vi "一体站流程自动启动.vi"(11 "参数":T1) -> ()   [LabVIEW 2016, in "PLC.lvlib"]
uses:
  PLC.lvlib
  <vilib>/ptbypt/NI_PtbyPt.lvlib
panel:
  out "s? t:f":enum16{"初始化", "采配水启动", "仪器操作", "反冲洗", "结束"}(ring)
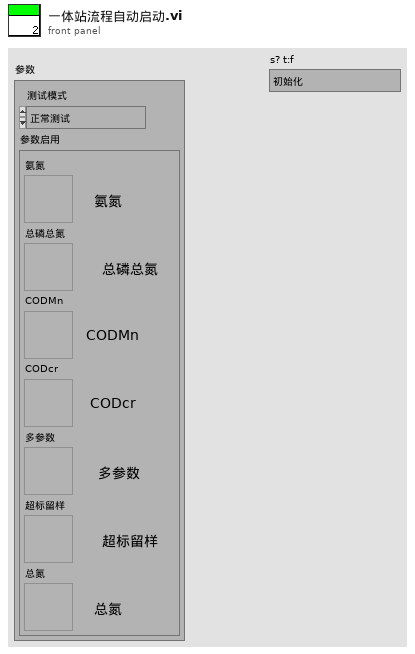
[diagram p1: front panel]
types:
  T1 = cluster{"测试模式":enum16{"正常测试", "集成干预"}, "参数启用":cluster{"氨氮":bool, "总磷总氮":bool, "CODMn":bool, "CODcr":bool, "多参数":bool, "超标留样":bool, "总氮":bool}}
  T2 = cluster{"命令":string, cluster{"starting address":u16, "holding register value":u16}}
  T3 = enum16{"启动测量", "标样核查", "零点核查", "跨度核查", "空白测试", "平行样测试", "加标回收", "空白校准", "标样校准", "初始化（清洗）", "停止测试", "仪器重启", "校时", "模式设置", "测量间隔设置"}
  T4 = cluster{"时间标识":timestamp, "设备":string, "日志信息":string, "流程参数":string}
  T5 = cluster{"测量模式":enum16{"水样测量", "标样核查", "零点核查", "跨度核查", "空白测试", "加标回收", "平行样", "校零", "校标"}}
  T6 = cluster{"时间标识":timestamp, "设备":string, "日志信息":string}
  T7 = enum16{"空闲", "水样测试", "标样核查", "零点核查", "跨度核查", "空白测试", "平行样测试", "加标回收", "空白校准", "标样校准", "初始化（清洗）"}
  T8 = enum32{"Bad", "Idle", "Run top level", "Running"}
  T9 = cluster{"R0":i16, "R1":i16, "R2":i16, "R3":i16, "R4":i16, "R5":i16, "R6":i16, "R7":i16, "R8":i16, "R9":i16, "R10":i16, "R11":i16, "R12":i16, "R13":i16, "R14":i16, "R15":i16, "R16":i16, "R17":i16, "R18":i16, "R19":i16, "R20":i16, "R21":i16, "R22":i16, "R23":i16, "R24":i16, "R25":i16, "R26":i16, "R27":i16, "R28":i16, "R29":i16, "R30":i16, "R31":i16, "R32":i16, "R33":i16, "R34":i16, "R35":i16, "R36":i16, "R37":i16, "R38":i16, "R39":i16, "R40":i16, "R41":i16, "R42":i16, "R43":i16, "R44":i16, "R45":i16, "R46":i16, "R47":i16, "R48":i16, "R49":i16, "R50":i16, "R51":i16, "R52":i16, "R53":i16, "R54":i16, "R55":i16, "R56":i16}
  T10 = cluster{"R100":i16, "R101":i16, "R102":i16, "R103":i16, "R104":i16, "R105":i16, "R106":i16, "R107":i16, "R108":i16, "R109":i16, "R110":i16, "R111":i16, "R112":i16, "R113":i16, "R114":i16, "R115":i16, "R116":i16, "R117":i16, "R118":i16, "R119":i16, "R120":i16, "R121":i16, "R122":i16, "R123":i16, "R124":i16}
  T11 = cluster{"氨氮":bool, "总磷总氮":bool, "CODmn":bool, "CODCr":bool, "多参数":bool, "超标留样":bool, "总氮":bool}
  T12 = cluster{"因子编码":u32, "单位":u16, "标样参考值":sgl, "水样数据时间":timestamp, "水样实测值":sgl, "水样数据标识":string, "标样数据时间":timestamp, "标样实测值":sgl, "标样数据标识":string, "空白数据时间":timestamp, "空白实测值":sgl, "空白数据标识":string, "零点核查数据时间":timestamp, "零点核查实测值":sgl, "零点核查数据标识":string, "跨度核查数据时间":timestamp, "跨度核查实测值":sgl, "跨度核查数据标识":string, "加标回收数据时间":timestamp, "加标回收实测值":sgl, "加标回收数据标识":string, "平行样数据时间":timestamp, "平行样实测值":sgl, "平行样数据标识":string, "F0":sgl, "F1":sgl, "F2":sgl, "F3":sgl, "F4":sgl, "F5":sgl, "F6":sgl, "F7":sgl, "温度":sgl, "湿度":sgl, "X值":sgl, "fidrange":u16}
  T13 = cluster{"COD浓度（mg/L)":dbl, "水样启动时间":timestamp, "加标回收启动时间":timestamp, "CODMn工作状态":enum16{"空闲", "水样测试", "标样核查", "零点核查", "跨度核查", "空白测试", "平行样测试", "加标回收", "空白校准", "标样校准", "初始化（清洗）"}, "多列列表框":i32}
  T14 = cluster{"因子编码":u32, "单位":u16, "标样参考值":sgl, "水样数据时间":timestamp, "水样实测值":sgl, "水样数据标识":string, "标样数据时间":timestamp, "标样实测值":sgl, "标样数据标识":string, "空白数据时间":timestamp, "空白实测值":sgl, "空白数据标识":string, "零点核查数据时间":timestamp, "零点核查实测值":sgl, "零点核查数据标识":string, "跨度核查数据时间":timestamp, "跨度核查实测值":sgl, "跨度核查数据标识":string, "加标回收数据时间":timestamp, "加标回收实测值":sgl, "加标回收数据标识":string, "平行样数据时间":timestamp, "平行样实测值":sgl, "平行样数据标识":string}
  T15 = cluster{"氨氮":bool, "总磷总氮":bool, "CODMn":bool, "CODcr":bool, "多参数":bool, "超标留样":bool, "总氮":bool}
  T16 = cluster{"时间标识":timestamp, "参数":string, "数据类型":string, "集成干预测试浓度值":dbl, "集成干预前测试时间":timestamp, "集成干预前测试浓度值":dbl}
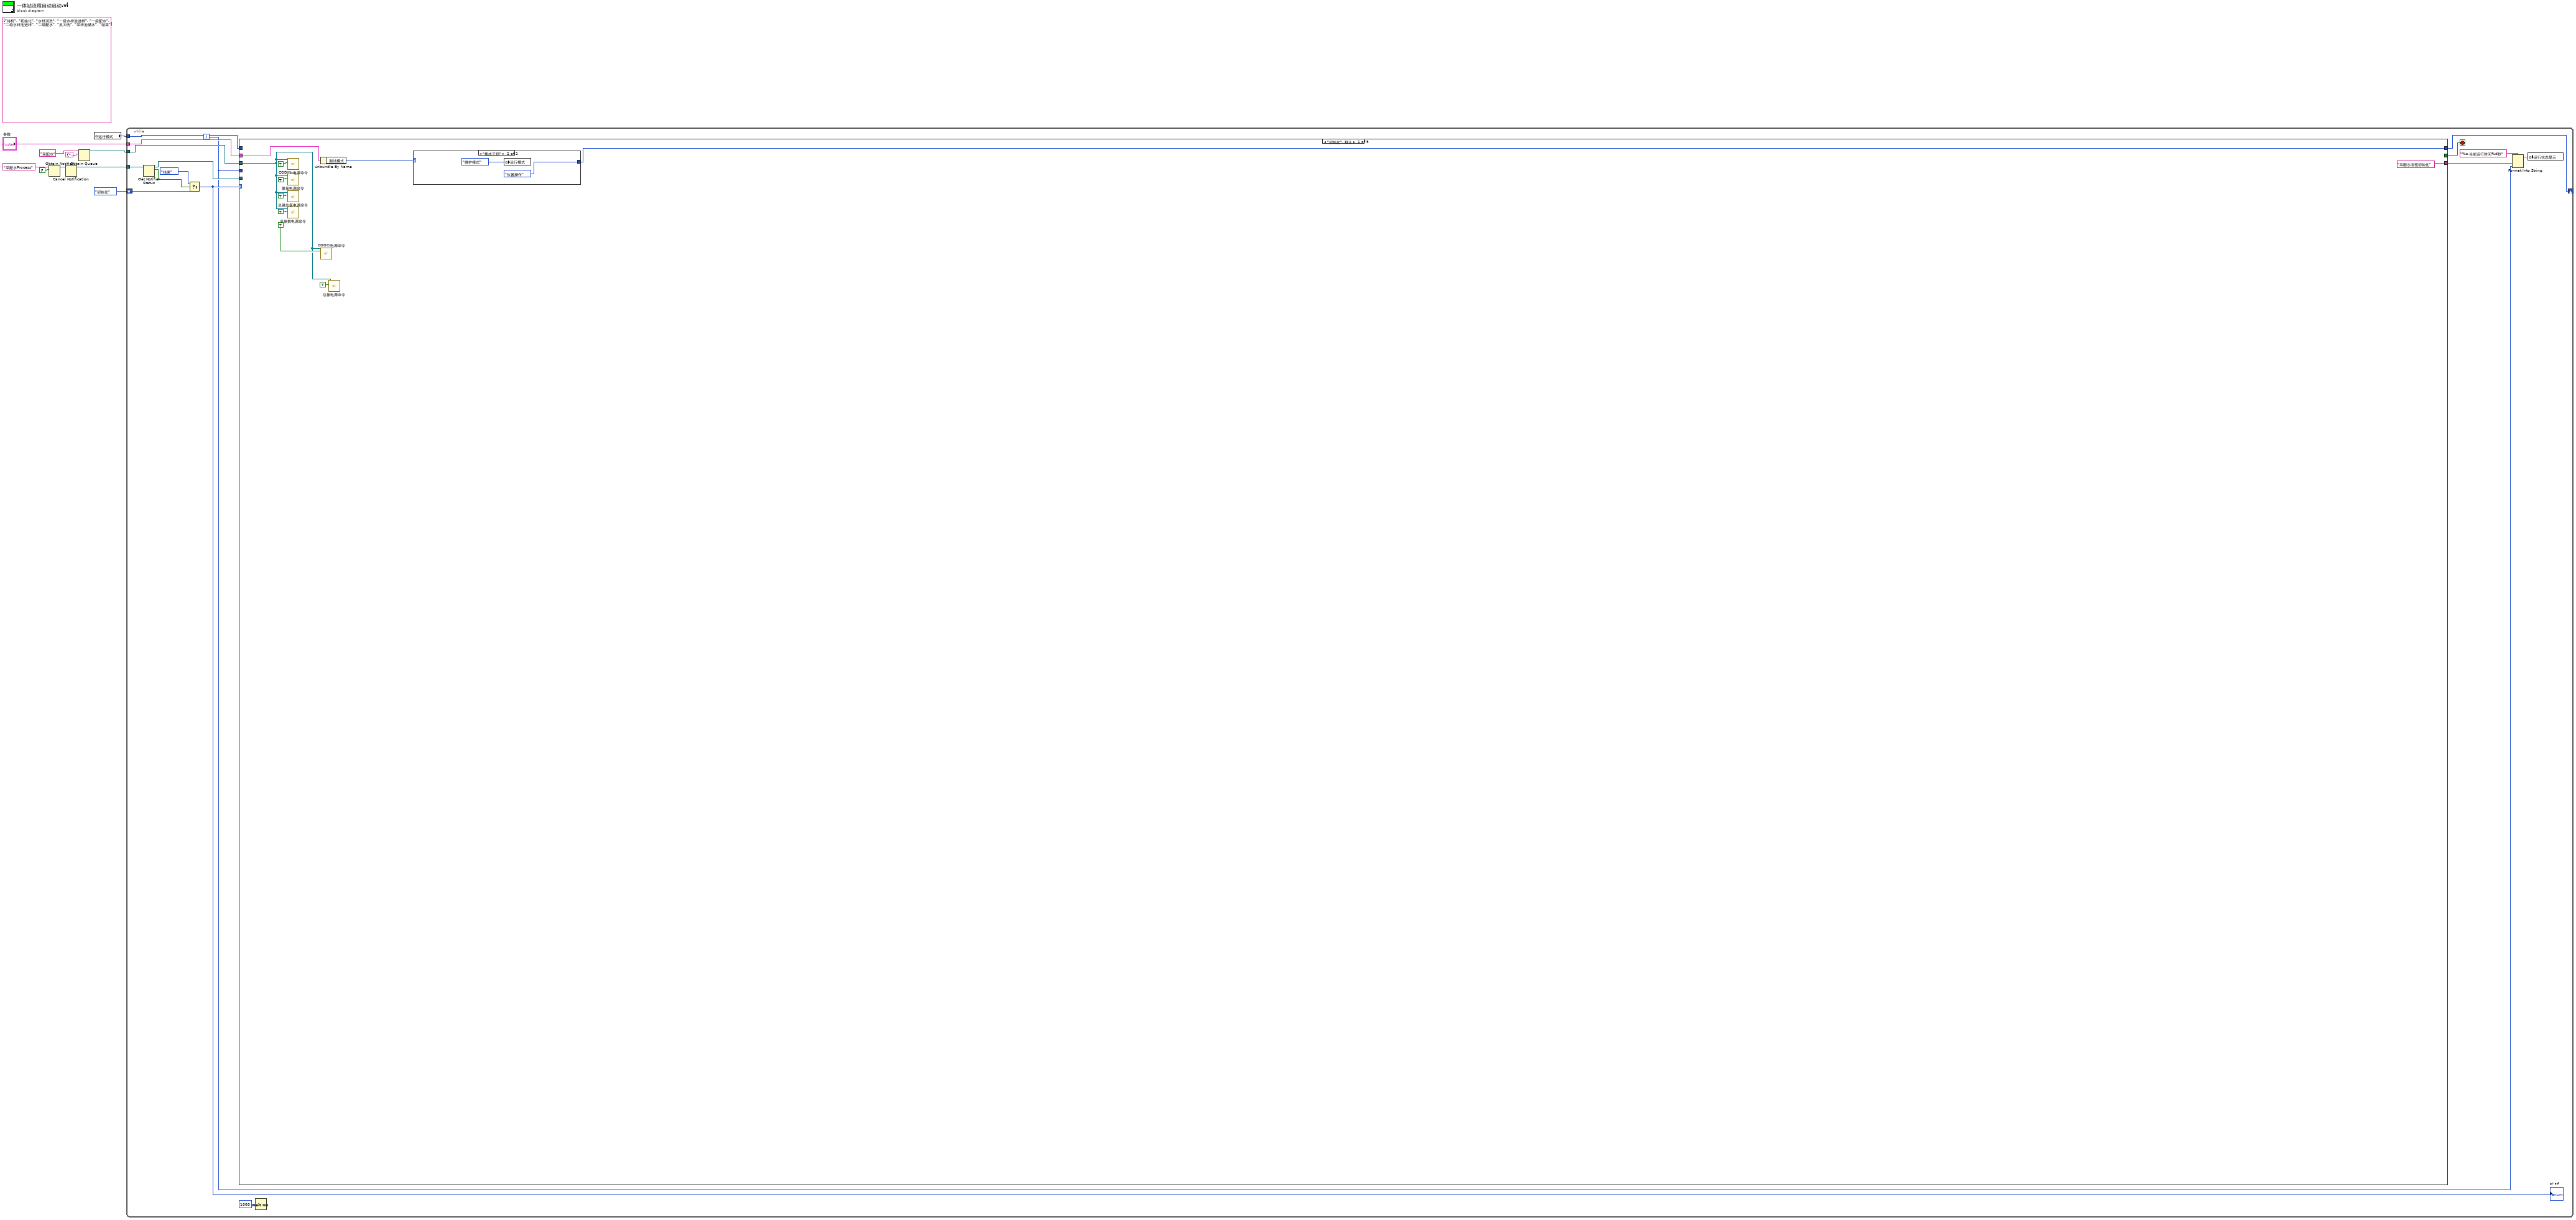
[diagram p0: block diagram]
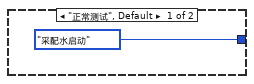
[diagram p2: hidden frame]
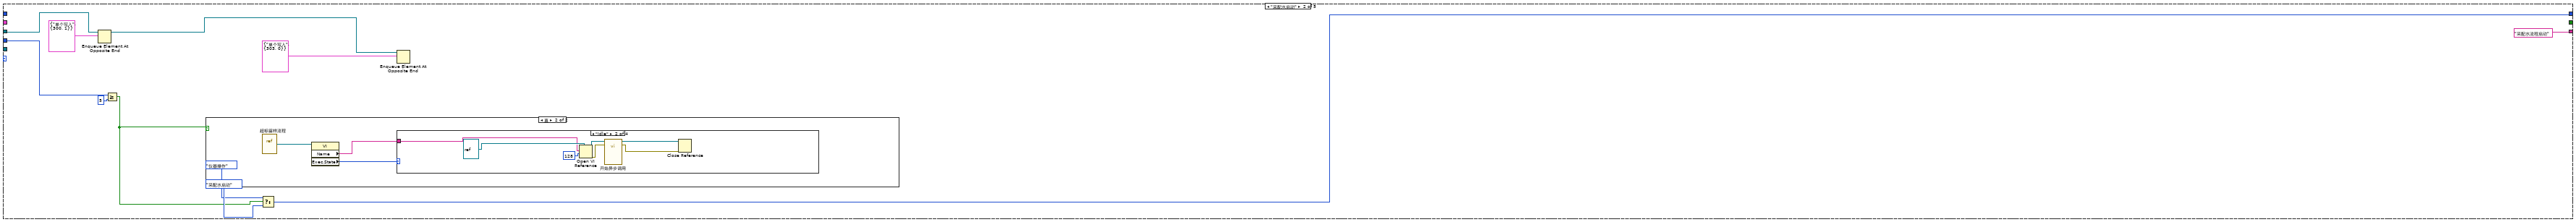
[diagram p3: hidden frame]
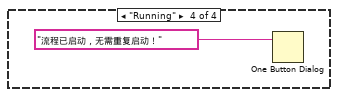
[diagram p7: hidden frame]
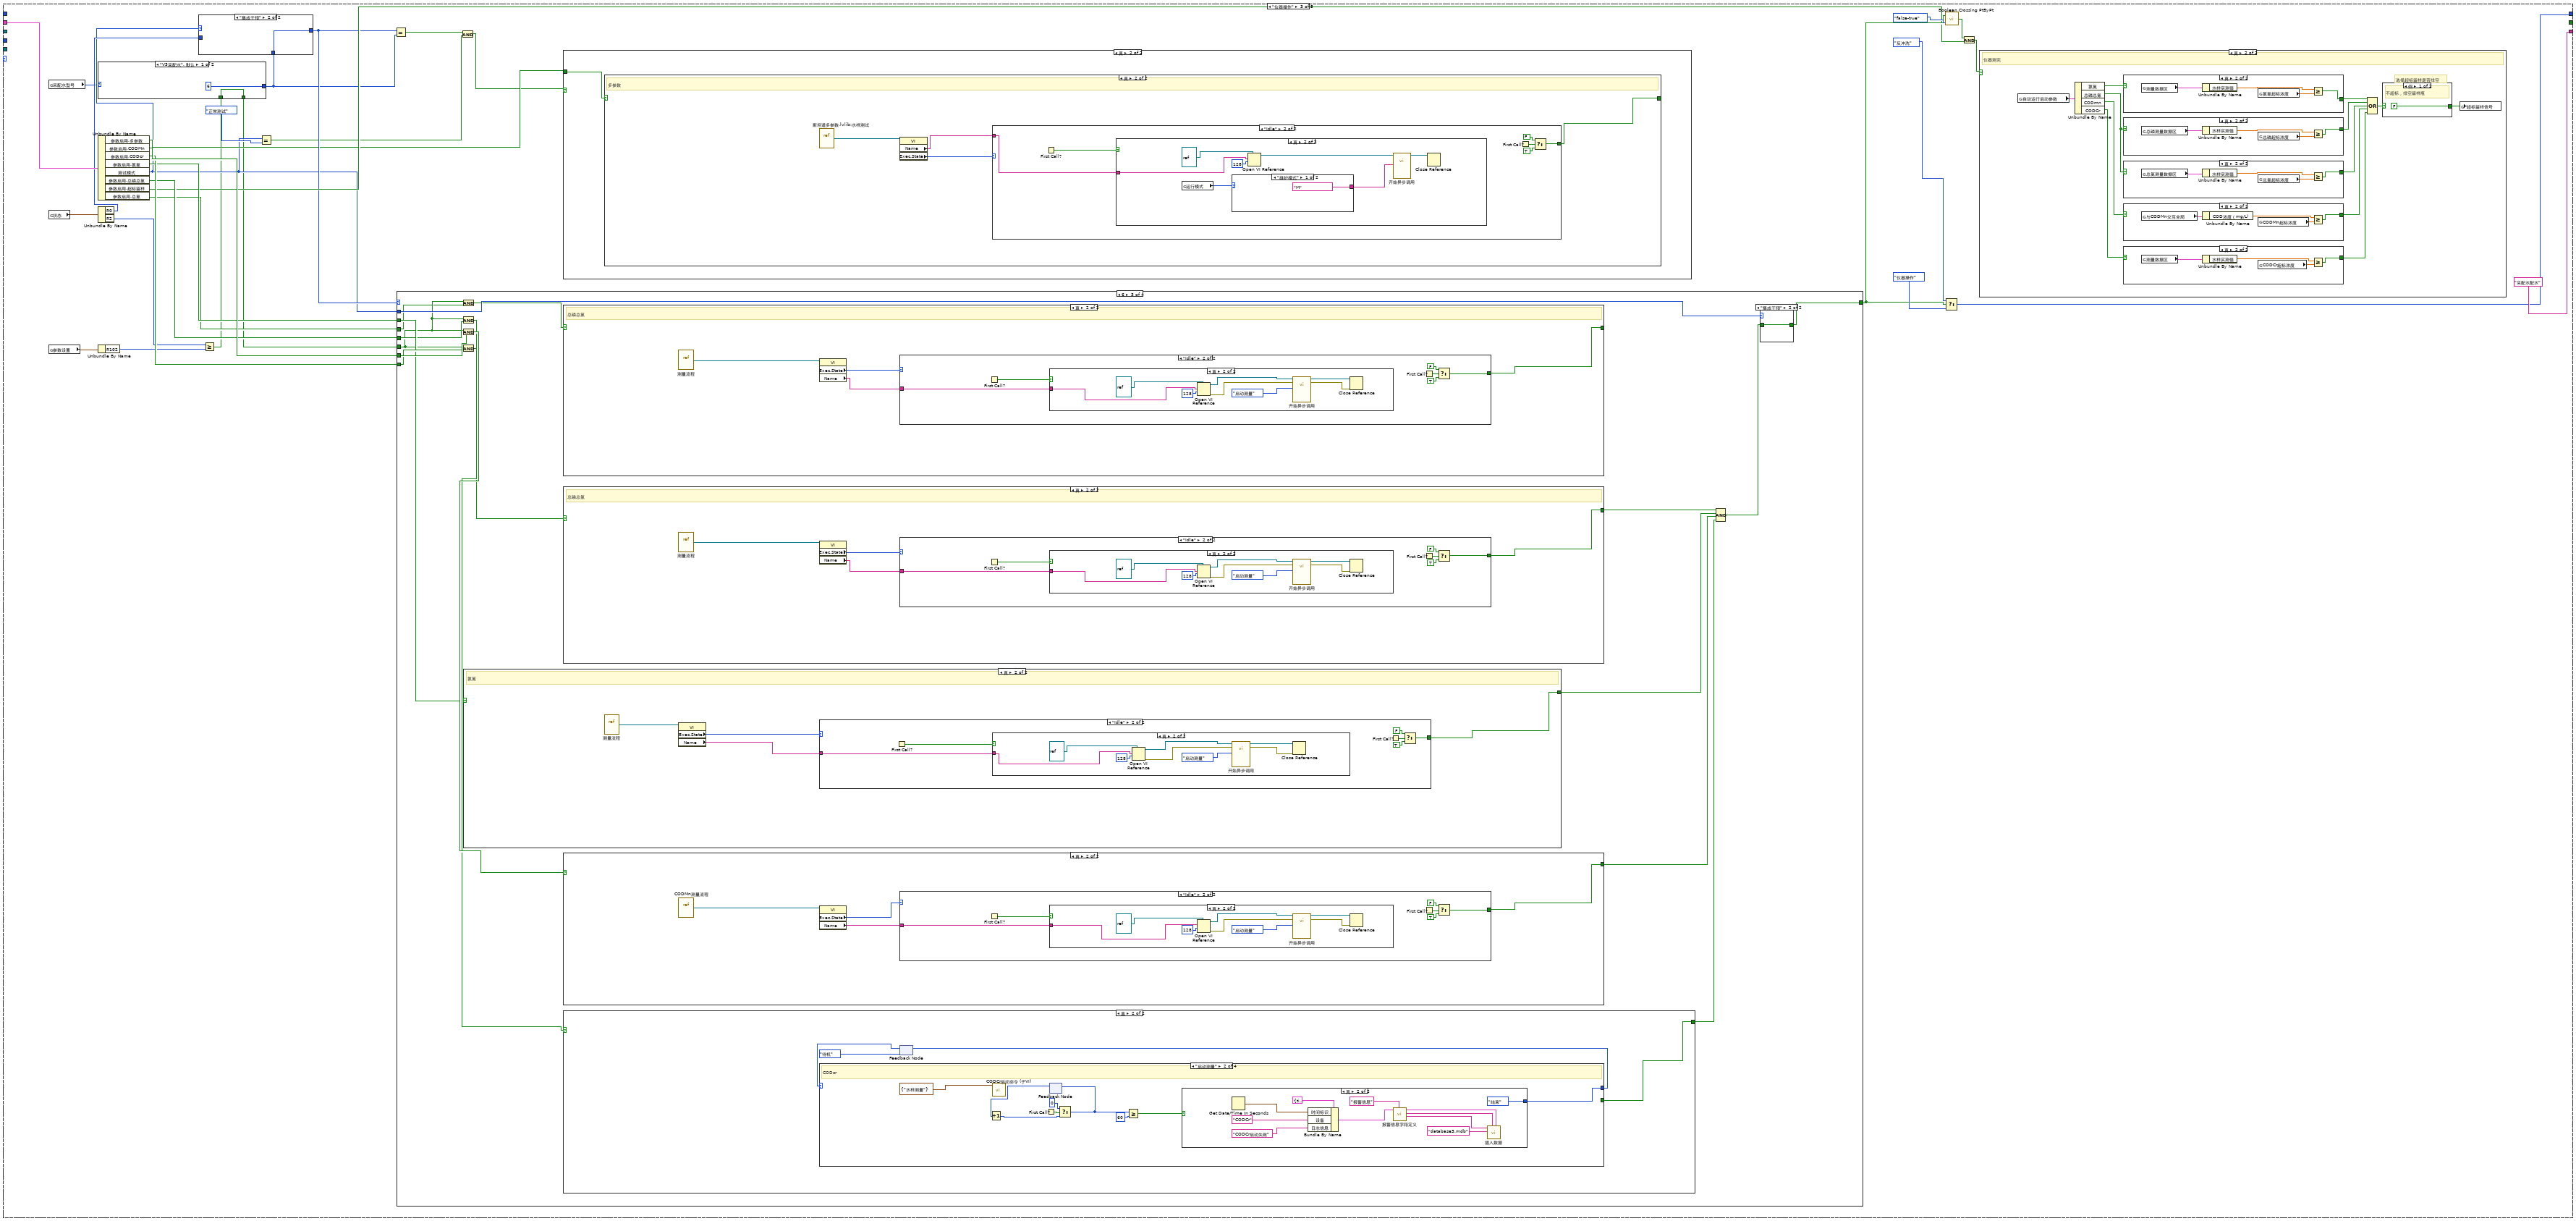
[diagram p8: hidden frame]
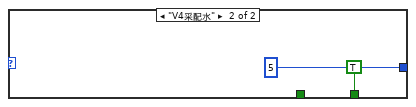
[diagram p9: hidden frame]
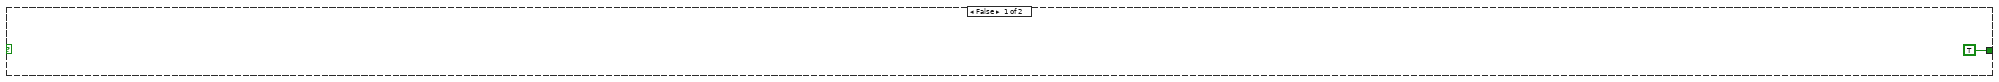
[diagram p11: hidden frame]
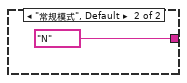
[diagram p14: hidden frame]
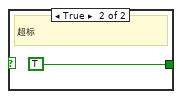
[diagram p16: hidden frame]
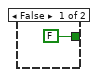
[diagram p17: hidden frame]
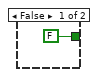
[diagram p18: hidden frame]
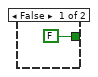
[diagram p19: hidden frame]
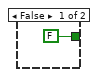
[diagram p20: hidden frame]
diagram:
  (unwired) string[][] [["待机"], ["初始化"], ["水样润洗"], ["一级水样池进样"], ["一级配水"], ["二级水样池进样"], ["二级配水"], ["反冲洗"], ["采样池储水"], ["结束"]] ("项名")
  n1 = Obtain Notifier(name (unnamed)="采配水Process" ("名称（未命名）"), notification data type=FALSE) -> (notifier out=w4:refnum<notifier>)  [unwired: 2 in, 2 out]
  n2 = Cancel Notification(0:w4) -> (8:w3:refnum<notifier>)  [unwired: 1 in, 2 out]
  n3 = Obtain Queue(name (unnamed)="采配水" ("名称（未命名）"), element data type=cluster{"命令":string, "数据":variant} {"命令"="", "数据"=variant}) -> (queue out=w7:refnum<queue>)  [unwired: 3 in, 2 out]
  n4 = global read "系统设置全局变量.vi" "运行模式"() -> (w1:enum16{"维护模式", "常规模式", "应急模式", "质控模式"})
  n5 = while {
    shift-right: [w23] -> _
    shift-left: enum16{"初始化", "采配水启动", "仪器操作", "反冲洗", "结束"}."初始化" ("枚举") -> [w19]
    tunnel: w7 -> [w26]
    tunnel: w3 -> [w22]
    tunnel: "参数" -> [w13]
    tunnel: w1 -> [w12]
    i -> [w11]
    stop <- w25 stop-if-true
    n6 = Get Notifier Status(notifier=w22) -> (notifier out=w14:refnum<notifier>, current notification=w21:bool)  [unwired: 1 in, 3 out]
    n7 = Select(t=enum16{"初始化", "采配水启动", "仪器操作", "反冲洗", "结束"}."结束" ("枚举"), s=w21, f=w19) -> (s? t:f=w18:enum16{"初始化", "采配水启动", "仪器操作", "反冲洗", "结束"})
    "s? t:f" <- w18
    n8 = case shown="\"初始化\", 默认" w18 {
      tunnel: w26 -> [w28 w51 _ _ w534]
      tunnel: [_ _ _ _ TRUE] -> w25
      tunnel: [w32 w44 w89 w318 enum16{"初始化", "采配水启动", "仪器操作", "反冲洗", "结束"}."结束" ("枚举")] -> w23
      tunnel: ["采配水流程初始化" "采配水流程启动" "采配水配水" "等待测试完成" "采配水结束"] -> w15
      tunnel: w14 -> [_ _ _ _ w535]
      tunnel: w13 -> [w30 _ w91 w317 w531]
      tunnel: w12 -> [_ _ _ w314 w530]
      tunnel: w11 -> [_ w49 _ _ _]
      frame "初始化", Default {
        n9 = call "CODMn电源命令.vi"("通电/断电"=TRUE, "队列"=w28) -> ()  [unwired: 9 in, 1 out]
        n10 = call "氨氮电源命令.vi"("通电/断电"=TRUE, "队列"=w28) -> ()  [unwired: 9 in, 1 out]
        n11 = call "总磷总氮电源命令.vi"("通电/断电"=TRUE, "队列"=w28) -> ()  [unwired: 9 in, 1 out]
        n12 = call "多参数电源命令.vi"("通电/断电"=TRUE, "队列"=w28) -> ()  [unwired: 9 in, 1 out]
        n13 = Unbundle By Name(w30) -> ("测试模式"=w29:enum16{"正常测试", "集成干预"})
        n14 = call "CODCr电源命令.vi"("通电/断电"=TRUE, "队列"=w28) -> ()  [unwired: 9 in, 1 out]
        n15 = call "总氮电源命令.vi"("通电/断电"=TRUE, "队列"=w28) -> ()  [unwired: 9 in, 1 out]
        n16 = case shown="\"集成干预\"" w29 {
          tunnel: [enum16{"初始化", "采配水启动", "仪器操作", "反冲洗", "结束"}."采配水启动" ("枚举") enum16{"初始化", "采配水启动", "仪器操作", "反冲洗", "结束"}."仪器操作" ("枚举")] -> w32
          frame "正常测试", Default {
          }
          frame "集成干预" {
            n17 = global write "系统设置全局变量.vi" "运行模式"(enum16{"维护模式", "常规模式", "应急模式", "质控模式"}."维护模式" ("运行模式")) -> ()
          }
        }
      }
      frame "采配水启动" {
        n18 = Enqueue Element At Opposite End(queue=w51, element=T2 {"命令"="单个写入", {"starting address"=300, "holding register value"=1}} ("元素")) -> (queue out=w42:refnum<queue>)  [unwired: 2 in, 2 out]
        n19 = Greater Or Equal?(x=w49, y=5) -> (x >= y?=w41:bool)
        n20 = case shown="真" w41 {
          frame False {
          }
          frame True {
            n21 = vi-ref "超标留样流程.vi"() -> (w54:refnum<vi>)
            n22 = property class="VI"(reference=w54) -> ("Name"=w53:string, "Exec.State"=w52:T8)  [unwired: 1 in, 2 out]
            n23 = case shown="\"Idle\"" w52 {
              tunnel: w53 -> [_ w57 _ _]
              frame "Bad", Default {
              }
              frame "Idle" {
                n24 = Open VI Reference(type specifier VI Refnum (for type only)=refnum<vi> refnum ("类型说明符VI引用句柄（仅用于类型）"), vi path=w57, options=128 ("选项")) -> (vi reference=w61:refnum<vi>, error out=w56:errorcluster)  [unwired: 3 in]
                n25 = call-by-ref "开始异步调用"(reference=w61, error in=w56) -> (reference out=w60:refnum<vi>, error out=w55:errorcluster)  [unwired: 12 in]
                n26 = Close Reference(reference=w60, error in (no error)=w55) -> ()  [unwired: 1 out]
              }
              frame "Run top level" {
              }
              frame "Running" {
                n27 = One Button Dialog(message="流程已启动，无需重复启动！" ("消息")) -> ()  [unwired: 1 in, 1 out]
              }
            }
          }
        }
        n28 = Select(t=enum16{"初始化", "采配水启动", "仪器操作", "反冲洗", "结束"}."仪器操作" ("枚举"), s=w41, f=enum16{"初始化", "采配水启动", "仪器操作", "反冲洗", "结束"}."采配水启动" ("枚举")) -> (s? t:f=w44:enum16{"初始化", "采配水启动", "仪器操作", "反冲洗", "结束"})
        n29 = Enqueue Element At Opposite End(queue=w42, element=T2 {"命令"="单个写入", {"starting address"=303, "holding register value"=0}} ("元素")) -> ()  [unwired: 2 in, 3 out]
      }
      frame "仪器操作" {
        n30 = global read "系统设置全局变量.vi" "采配水型号"() -> (w64:enum16{"V3采配水", "V4采配水"})
        n31 = global read "采配水全局变量.vi" "状态"() -> (w93:T9)
        n32 = global read "采配水全局变量.vi" "参数设置"() -> (w82:T10)
        n33 = Unbundle By Name(w91) -> ("参数启用.多参数"=w72:bool, "参数启用.CODMn"=w87:bool, "参数启用.CODcr"=w86:bool, "参数启用.氨氮"=w85:bool, "测试模式"=w68:enum16{"正常测试", "集成干预"}, "参数启用.总磷总氮"=w80:bool, "参数启用.超标留样"=w75:bool, "参数启用.总氮"=w67:bool)
        n34 = Unbundle By Name(w93) -> ("R0"=w84:i16, "R2"=w81:i16)
        n35 = Unbundle By Name(w82) -> ("R102"=w83:i16)
        n36 = Greater Or Equal?(x=w81, y=w83) -> (x >= y?=w66:bool)
        n37 = case shown="\"V3采配水\", 默认" w64 {
          tunnel: [6 5] -> w63
          tunnel: w66 -> [w94 _]
          tunnel: [w94 TRUE] -> w65
          frame "V3采配水", Default {
          }
          frame "V4采配水" {
          }
        }
        n38 = case shown="\"集成干预\"" w68 {
          tunnel: w84 -> [w158 _]
          tunnel: [w158 w159] -> w74
          tunnel: w63 -> [_ w159]
          frame "正常测试", Default {
          }
          frame "集成干预" {
          }
        }
        n39 = Equal?(x=w68, y=enum16{"正常测试", "集成干预"}."正常测试") -> (x = y?=w69:bool)
        n40 = Equal?(x=w74, y=w63) -> (x = y?=w73:bool)
        n41 = case shown="6" w74 {
          tunnel: [w161 _ w174 TRUE] -> w76
          tunnel: w87 -> [_ _ w183 _]
          tunnel: w86 -> [_ _ w180 _]
          tunnel: w85 -> [_ _ w179 _]
          tunnel: w65 -> [_ _ w169 _]
          tunnel: w68 -> [_ _ w170 _]
          tunnel: w80 -> [_ _ w173 _]
          tunnel: w67 -> [_ _ w168 _]
          frame 0, Default {
            n42 = global read "采配水全局变量.vi" "状态"() -> (w164:T9)
            n43 = global read "采配水全局变量.vi" "报警簇"() -> (w165:bool[])
            n44 = Unbundle By Name(w164) -> ("R0"=w163:i16)
            n45 = Index Array(array=w165, index=0 ("索引")) -> (element=w160:bool)
            n46 = Equal To 0?(x=w163) -> (x = 0?=w166:bool)
            n47 = Compound Arithmetic op=OR ("复合运算")(w166, w160) -> (w161:bool)
          }
          frame 5 {
          }
          frame 6 {
            n48 = And(x=w169, y=w168) -> (x .and. y?=w167:bool)
            n49 = And(x=w169, y=w173) -> (x .and. y?=w172:bool)
            n50 = And(x=w169, y=w183) -> (x .and. y?=w182:bool)
            n51 = And(x=w169, y=w180) -> (x .and. y?=w181:bool)
            n52 = case "条件结构" shown="真" w179 {
              tunnel: [TRUE ("t") w227] -> w178
              frame False {
              }
              frame True {
                # "氨氮"
                n53 = vi-ref "测量流程.vi"() -> (w226:refnum<vi>)
                n54 = property class="VI"(reference=w226) -> ("Exec.State"=w225:T8, "Name"=w224:string)  [unwired: 1 in, 2 out]
                n55 = case shown="\"Idle\"" w225 {
                  tunnel: w224 -> [_ w233]
                  tunnel: [_ w228] -> w227
                  frame "Bad", Default {
                  }
                  frame "Idle" {
                    n56 = First Call?() -> (First Call?: T/F=w232:bool)
                    n57 = case shown="真" w232 {
                      tunnel: w233 -> [_ w238]
                      frame False {
                      }
                      frame True {
                        n58 = Open VI Reference(type specifier VI Refnum (for type only)=refnum<vi> refnum, vi path=w238, options=128 ("选项")) -> (vi reference=w236:refnum<vi>, error out=w239:errorcluster)  [unwired: 3 in]
                        n59 = call-by-ref "开始异步调用"(reference=w236, error in=w239, "控制命令"=T3."启动测量") -> (reference out=w240:refnum<vi>, error out=w241:errorcluster)  [unwired: 11 in]
                        n60 = Close Reference(reference=w240, error in (no error)=w241) -> ()  [unwired: 1 out]
                      }
                    }
                    n61 = First Call?() -> (First Call?: T/F=w231:bool)
                    n62 = Select(t=FALSE, s=w231, f=TRUE) -> (s? t:f=w228:bool)
                  }
                }
              }
            }
            n63 = case "条件结构" shown="真" w167 {
              tunnel: [TRUE ("t") w188] -> _
              frame False {
              }
              frame True {
                # "总磷总氮"
                n64 = vi-ref "测量流程.vi"() -> (w187:refnum<vi>)
                n65 = property class="VI"(reference=w187) -> ("Exec.State"=w186:T8, "Name"=w185:string)  [unwired: 1 in, 2 out]
                n66 = case shown="\"Idle\"" w186 {
                  tunnel: w185 -> [_ w194]
                  tunnel: [_ w189] -> w188
                  frame "Bad", Default {
                  }
                  frame "Idle" {
                    n67 = First Call?() -> (First Call?: T/F=w193:bool)
                    n68 = case shown="真" w193 {
                      tunnel: w194 -> [_ w199]
                      frame False {
                      }
                      frame True {
                        n69 = Open VI Reference(type specifier VI Refnum (for type only)=refnum<vi> refnum, vi path=w199, options=128 ("选项")) -> (vi reference=w197:refnum<vi>, error out=w200:errorcluster)  [unwired: 3 in]
                        n70 = call-by-ref "开始异步调用"(reference=w197, error in=w200, "控制命令"=T3."启动测量") -> (reference out=w201:refnum<vi>, error out=w202:errorcluster)  [unwired: 11 in]
                        n71 = Close Reference(reference=w201, error in (no error)=w202) -> ()  [unwired: 1 out]
                      }
                    }
                    n72 = First Call?() -> (First Call?: T/F=w192:bool)
                    n73 = Select(t=FALSE, s=w192, f=TRUE) -> (s? t:f=w189:bool)
                  }
                }
              }
            }
            n74 = case "条件结构" shown="真" w172 {
              tunnel: [TRUE ("t") w207] -> w171
              frame False {
              }
              frame True {
                # "总磷总氮"
                n75 = vi-ref "测量流程.vi"() -> (w206:refnum<vi>)
                n76 = property class="VI"(reference=w206) -> ("Exec.State"=w205:T8, "Name"=w204:string)  [unwired: 1 in, 2 out]
                n77 = case shown="\"Idle\"" w205 {
                  tunnel: w204 -> [_ w213]
                  tunnel: [_ w208] -> w207
                  frame "Bad", Default {
                  }
                  frame "Idle" {
                    n78 = First Call?() -> (First Call?: T/F=w212:bool)
                    n79 = case shown="真" w212 {
                      tunnel: w213 -> [_ w218]
                      frame False {
                      }
                      frame True {
                        n80 = Open VI Reference(type specifier VI Refnum (for type only)=refnum<vi> refnum, vi path=w218, options=128 ("选项")) -> (vi reference=w216:refnum<vi>, error out=w219:errorcluster)  [unwired: 3 in]
                        n81 = call-by-ref "开始异步调用"(reference=w216, error in=w219, "控制命令"=T3."启动测量") -> (reference out=w220:refnum<vi>, error out=w221:errorcluster)  [unwired: 11 in]
                        n82 = Close Reference(reference=w220, error in (no error)=w221) -> ()  [unwired: 1 out]
                      }
                    }
                    n83 = First Call?() -> (First Call?: T/F=w211:bool)
                    n84 = Select(t=FALSE, s=w211, f=TRUE) -> (s? t:f=w208:bool)
                  }
                }
              }
            }
            n85 = case shown="真" w182 {
              tunnel: [TRUE w298] -> w177
              frame False {
              }
              frame True {
                n86 = vi-ref "CODMn测量流程.vi"() -> (w295:refnum<vi>)
                n87 = property class="VI"(reference=w295) -> ("Exec.State"=w296:T8, "Name"=w297:string)  [unwired: 1 in, 2 out]
                n88 = case shown="\"Idle\"" w296 {
                  tunnel: w297 -> [_ w304]
                  tunnel: [_ w299] -> w298
                  frame "Bad", Default {
                  }
                  frame "Idle" {
                    n89 = First Call?() -> (First Call?: T/F=w303:bool)
                    n90 = case shown="真" w303 {
                      tunnel: w304 -> [_ w309]
                      frame False {
                      }
                      frame True {
                        n91 = Open VI Reference(type specifier VI Refnum (for type only)=refnum<vi> refnum, vi path=w309, options=128 ("选项")) -> (vi reference=w307:refnum<vi>, error out=w310:errorcluster)  [unwired: 3 in]
                        n92 = call-by-ref "开始异步调用"(reference=w307, error in=w310, "控制命令"=T3."启动测量") -> (reference out=w311:refnum<vi>, error out=w312:errorcluster)  [unwired: 11 in]
                        n93 = Close Reference(reference=w311, error in (no error)=w312) -> ()  [unwired: 1 out]
                      }
                    }
                    n94 = First Call?() -> (First Call?: T/F=w302:bool)
                    n95 = Select(t=FALSE, s=w302, f=TRUE) -> (s? t:f=w299:bool)
                  }
                }
              }
            }
            n96 = case shown="真" w181 {
              tunnel: [TRUE w246] -> w176
              frame False {
              }
              frame True {
                n97 = feedback #1(enum16{"待机", "启动测量", "测量中", "结束"}."待机") -> (w244:enum16{"待机", "启动测量", "测量中", "结束"})
                n98 = case shown="\"启动测量\"" w244 {
                  tunnel: [enum16{"待机", "启动测量", "测量中", "结束"}."启动测量" w261 w281 enum16{"待机", "启动测量", "测量中", "结束"}."结束"] -> w243
                  tunnel: [_ _ _ TRUE] -> w246
                  frame "待机", Default {
                    n99 = Get Date/Time In Seconds() -> (seconds since 1Jan1904=w251:timestamp)
                    n100 = Bundle By Name(cluster=T4 {"时间标识"=timestamp(0 s since 1904-01-01), "设备"="", "日志信息"="", "流程参数"=""} ("data in"), "时间标识"=w251, "设备"="CODCr", "日志信息"="-->>CODCr启动") -> (w247:T4)
                    n101 = call "总磷总氮操作日志.vi"("data in"=w247) -> ()  [unwired: 11 in]
                  }
                  frame "启动测量" {
                    # "CODcr"
                    n102 = call "CODCr启动命令 (子VI).vi"("启动测量模式"=T5 {"测量模式"=enum."水样测量"}) -> ()  [unwired: 11 in]
                    n103 = First Call?() -> (First Call?: T/F=w256:bool)
                    n104 = feedback #2() -> (w257:i32)  [unwired: 1 in]
                    n105 = Increment(x=w257) -> (x+1=w258:i32)
                    n106 = Select(t=0, s=w256, f=w258) -> (s? t:f=w259:i32)
                    n107 = feedback-in #2(w259) -> ()
                    n108 = Greater Or Equal?(x=w259, y=60) -> (x >= y?=w254:bool)
                    n109 = case shown="真" w254 {
                      tunnel: [w262 enum16{"待机", "启动测量", "测量中", "结束"}."结束"] -> w261
                      frame False {
                        n110 = global read "CODcr全局变量.vi" "工作状态"() -> (w263:T7)
                        n111 = Not Equal To 0?(x=w263) -> (x != 0?=w264:bool)
                        n112 = Select(t=enum16{"待机", "启动测量", "测量中", "结束"}."测量中", s=w264, f=enum16{"待机", "启动测量", "测量中", "结束"}."启动测量") -> (s? t:f=w262:enum16{"待机", "启动测量", "测量中", "结束"})
                      }
                      frame True {
                        n113 = Get Date/Time In Seconds() -> (seconds since 1Jan1904=w273:timestamp)
                        n114 = Bundle By Name(cluster=T6 {"时间标识"=timestamp(0 s since 1904-01-01), "设备"="", "日志信息"=""} ("data in"), "时间标识"=w273, "设备"="CODCr", "日志信息"="CODCr启动失败") -> (w267:T6)
                        n115 = call "报警信息字段定义.vi"("table输入"="报警信息", "data in"=w267) -> ("table输出"=w270:string, "columns"=w271:string[], "data out"=w272:T6)  [unwired: 7 in]
                        n116 = call "插入数据.vi"("data"=w272, "columns"=w271, "database"="database3.mdb", "table"=w270) -> ()  [unwired: 7 in, 1 out]
                      }
                    }
                  }
                  frame "测量中" {
                    n117 = global read "CODcr全局变量.vi" "工作状态"() -> (w280:T7)
                    n118 = Equal?(x=w280, y=T7."空闲" ("工作状态")) -> (x = y?=w279:bool)
                    n119 = case shown="假" w279 {
                      tunnel: [w282 enum16{"待机", "启动测量", "测量中", "结束"}."结束"] -> w281
                      frame False {
                        n120 = flat-sequence {
                          tunnel: [enum16{"待机", "启动测量", "测量中", "结束"}."测量中"] -> w282
                          frame #0 {
                            n121 = Wait (ms)(milliseconds to wait=u32 1000 ("等待时间（毫秒）")) -> ()  [unwired: 1 out]
                          }
                          frame #1 {
                          }
                        }
                      }
                      frame True {
                      }
                    }
                  }
                  frame "结束" {
                    n122 = First Call?() -> (First Call?: T/F=w286:bool)
                    n123 = case shown="真" w286 {
                      frame False {
                      }
                      frame True {
                        n124 = Get Date/Time In Seconds() -> (seconds since 1Jan1904=w293:timestamp)
                        n125 = Bundle By Name(cluster=T4 {"时间标识"=timestamp(0 s since 1904-01-01), "设备"="", "日志信息"="", "流程参数"=""} ("data in"), "时间标识"=w293, "设备"="CODCr", "日志信息"="-->>CODCr停止") -> (w289:T4)
                        n126 = call "总磷总氮操作日志.vi"("data in"=w289) -> ()  [unwired: 11 in]
                      }
                    }
                  }
                }
                n127 = feedback-in #1(w243) -> ()
              }
            }
            n128 = Compound Arithmetic op=AND ("复合运算")(w171, w178, w177, w176) -> (w175:bool)
            n129 = case shown="\"集成干预\"" w170 {
              tunnel: w175 -> [_ w222]
              tunnel: [_ w222] -> w174
              frame "正常测试", Default {
              }
              frame "集成干预" {
              }
            }
          }
          frame 7..9 {
          }
        }
        n130 = And(x=w73, y=w69) -> (x .and. y?=w70:bool)
        n131 = case shown="真" w70 {
          tunnel: w72 -> [_ w98]
          frame False {
          }
          frame True {
            n132 = case shown="真" w98 {
              tunnel: [TRUE ("t") w103] -> _
              frame False {
              }
              frame True {
                # "多参数"
                n133 = vi-ref "斯坦道多参数.lvlib:水样测试.vi"() -> (w101:refnum<vi>)
                n134 = property class="VI"(reference=w101) -> ("Name"=w100:string, "Exec.State"=w102:T8)  [unwired: 1 in, 2 out]
                n135 = case shown="\"Idle\"" w102 {
                  tunnel: w100 -> [_ w109]
                  tunnel: [_ w104] -> w103
                  frame "Bad", Default {
                  }
                  frame "Idle" {
                    n136 = First Call?() -> (First Call?: T/F=w108:bool)
                    n137 = case shown="真" w108 {
                      tunnel: w109 -> [_ w115]
                      frame False {
                      }
                      frame True {
                        n138 = global read "系统设置全局变量.vi" "运行模式"() -> (w112:enum16{"维护模式", "常规模式", "应急模式", "质控模式"})
                        n139 = case shown="\"维护模式\"" w112 {
                          tunnel: ["M" ("数据标记表") "N" ("数据标记表")] -> w111
                          frame "维护模式" {
                          }
                          frame "常规模式", Default {
                          }
                        }
                        n140 = Open VI Reference(type specifier VI Refnum (for type only)=refnum<vi> refnum, vi path=w115, options=128 ("选项")) -> (vi reference=w114:refnum<vi>)  [unwired: 3 in, 1 out]
                        n141 = call-by-ref "开始异步调用"(reference=w114, "数据标记表"=w111) -> (reference out=w113:refnum<vi>)  [unwired: 12 in, 1 out]
                        n142 = Close Reference(reference=w113) -> ()  [unwired: 1 in, 1 out]
                      }
                    }
                    n143 = First Call?() -> (First Call?: T/F=w107:bool)
                    n144 = Select(t=FALSE, s=w107, f=TRUE) -> (s? t:f=w104:bool)
                  }
                }
              }
            }
          }
        }
        n145 = Select(t=enum16{"初始化", "采配水启动", "仪器操作", "反冲洗", "结束"}."反冲洗" ("枚举"), s=w76, f=enum16{"初始化", "采配水启动", "仪器操作", "反冲洗", "结束"}."仪器操作" ("枚举")) -> (s? t:f=w89:enum16{"初始化", "采配水启动", "仪器操作", "反冲洗", "结束"})
        n146 = call <vilib>:"Boolean Crossing PtByPt.vi"("direction"=enum16{"either", "false-true", "true-false"}."false-true", "input"=w76) -> ("crossing"=w78:bool)  [unwired: 1 in]
        n147 = And(x=w78, y=w75) -> (x .and. y?=w77:bool)
        n148 = case shown="真" w77 {
          frame False {
          }
          frame True {
            # "选择超标留样是否排空"
            # "仪器测完"
            n149 = global read "系统设置全局变量.vi" "自动运行启动参数"() -> (w123:T11)
            n150 = Unbundle By Name(w123) -> ("氨氮"=w122:bool, "总磷总氮"=w121:bool, "CODmn"=w120:bool, "CODCr"=w119:bool)
            n151 = case shown="真" w122 {
              tunnel: [FALSE w156] -> w130
              frame False {
              }
              frame True {
                n152 = global read "VAR总磷总氮全局变量.vi" "测量数据区"() -> (w155:T12)
                n153 = Unbundle By Name(w155) -> ("水样实测值"=w157:sgl)
                n154 = global read "外部交互全局.vi" "氨氮超标浓度"() -> (w154:dbl)
                n155 = Greater Or Equal?(x=w157, y=w154) -> (x >= y?=w156:bool)
              }
            }
            n156 = case shown="真" w121 {
              tunnel: [FALSE w152] -> w129
              frame False {
              }
              frame True {
                n157 = global read "VAR总磷总氮全局变量.vi" "总磷测量数据区"() -> (w149:T12)
                n158 = Unbundle By Name(w149) -> ("水样实测值"=w151:sgl)
                n159 = global read "外部交互全局.vi" "总磷超标浓度"() -> (w150:dbl)
                n160 = Greater Or Equal?(x=w151, y=w150) -> (x >= y?=w152:bool)
              }
            }
            n161 = case shown="真" w121 {
              tunnel: [FALSE w147] -> w128
              frame False {
              }
              frame True {
                n162 = global read "VAR总磷总氮全局变量.vi" "总氮测量数据区"() -> (w144:T12)
                n163 = Unbundle By Name(w144) -> ("水样实测值"=w146:sgl)
                n164 = global read "外部交互全局.vi" "总氮超标浓度"() -> (w145:dbl)
                n165 = Greater Or Equal?(x=w146, y=w145) -> (x >= y?=w147:bool)
              }
            }
            n166 = case shown="真" w120 {
              tunnel: [FALSE w142] -> w127
              frame False {
              }
              frame True {
                n167 = global read "modbus slave全局.vi" "与CODMn交互全局"() -> (w140:T13)
                n168 = Unbundle By Name(w140) -> ("COD浓度（mg/L)"=w139:dbl)
                n169 = global read "外部交互全局.vi" "CODMn超标浓度"() -> (w141:dbl)
                n170 = Greater Or Equal?(x=w139, y=w141) -> (x >= y?=w142:bool)
              }
            }
            n171 = case shown="真" w119 {
              tunnel: [FALSE w137] -> w126
              frame False {
              }
              frame True {
                n172 = global read "CODcr全局变量.vi" "测量数据区"() -> (w134:T14)
                n173 = Unbundle By Name(w134) -> ("水样实测值"=w136:sgl)
                n174 = global read "外部交互全局.vi" "CODCr超标浓度"() -> (w135:dbl)
                n175 = Greater Or Equal?(x=w136, y=w135) -> (x >= y?=w137:bool)
              }
            }
            n176 = Compound Arithmetic op=OR ("复合运算")(w130, w129, w128, w127, w126) -> (w125:bool)
            n177 = case shown="假" w125 {
              tunnel: [FALSE ("超标留样信号") TRUE ("超标留样信号")] -> w124
              frame False {
                # "不超标，排空留样瓶"
              }
              frame True {
                # "超标"
              }
            }
            n178 = global write "外部交互全局.vi" "超标留样信号"(w124) -> ()
          }
        }
      }
      frame "反冲洗" {
        n179 = First Call?() -> (First Call?: T/F=w315:bool)
        n180 = global read "采配水全局变量.vi" "状态"() -> (w323:T9)
        n181 = case shown="真" w315 {
          tunnel: w317 -> [_ w327]
          tunnel: w314 -> [_ w324]
          frame False {
          }
          frame True {
            n182 = Unbundle By Name(w327) -> ("测试模式"=w326:enum16{"正常测试", "集成干预"}, "参数启用"=w325:T15)
            n183 = case shown="\"正常测试\", 默认" w326 {
              tunnel: w325 -> [w336 w447]
              tunnel: w324 -> [_ w441]
              frame "正常测试", Default {
                n184 = global read "系统设置全局变量.vi" "运行模式"() -> (w334:enum16{"维护模式", "常规模式", "应急模式", "质控模式"})
                n185 = global read "采配水全局变量.vi" "报警簇"() -> (w341:bool[])
                n186 = global read "采配水全局变量.vi" "输入状态"() -> (w333:bool[])
                n187 = case shown="\"维护模式\"" w334 {
                  tunnel: ["M" ("table") "N" ("table")] -> w335
                  frame "维护模式" {
                  }
                  frame "常规模式", Default {
                  }
                }
                n188 = Index Array(array=w333, index=7 ("索引")) -> (element=w331:bool)
                n189 = Index Array(array=w341, index #1=0 ("索引"), index #2=11 ("索引")) -> (element #1=w338:bool, element #2=w337:bool)
                n190 = Select(t="P" ("数据标识"), s=w331, f="Z" ("数据标识")) -> (s? t:f=w328:string)
                n191 = case shown="真" w338 {
                  tunnel: w337 -> [w347 w355]
                  tunnel: w336 -> [w346 w365]
                  tunnel: w335 -> [w344 w358]
                  tunnel: w328 -> [_ w357]
                  frame False {
                    n192 = Unbundle By Name(w346) -> ("氨氮"=w345:bool)
                    n193 = case shown="真" w347 {
                      tunnel: w345 -> [_ w349]
                      tunnel: w344 -> [_ w348]
                      frame False {
                      }
                      frame True {
                        n194 = case shown="真" w349 {
                          tunnel: w348 -> [_ w350]
                          tunnel: [_ w351] -> _
                          frame False {
                          }
                          frame True {
                            n195 = call "取水点无水样数据存储.vi"("数据标识"="lw", "数据类型"=w350, "table"="氨氮") -> ("error out"=w351:errorcluster)  [unwired: 8 in]
                          }
                        }
                      }
                    }
                  }
                  frame True {
                    n196 = Unbundle By Name(w365) -> ("氨氮"=w364:bool, "CODMn"=w363:bool, "CODcr"=w362:bool, "多参数"=w361:bool, "总磷总氮"=w360:bool, "总氮"=w359:bool)
                    n197 = Not(x=w355) -> (.not. x?=w354:bool)
                    n198 = And(x=w361, y=w354) -> (x .and. y?=w356:bool)
                    n199 = case shown="真" w364 {
                      tunnel: w358 -> [_ w432]
                      tunnel: w357 -> [_ w431]
                      tunnel: [_ w430] -> _
                      frame False {
                      }
                      frame True {
                        n200 = global read "系统设置全局变量.vi" "营养盐类型"() -> (w429:enum16{"氨氮、总磷总氮", "氨氮总磷", "氨氮、总磷、总氮"})
                        n201 = call "取水点无水样数据存储.vi"("数据标识"=w431, "数据类型"=w432, "table"="氨氮") -> ("error out"=w433:errorcluster)  [unwired: 8 in]
                        n202 = case shown="\"氨氮总磷\"" w429 {
                          tunnel: w433 -> [_ w438]
                          tunnel: w432 -> [_ w437]
                          tunnel: w431 -> [_ w436]
                          tunnel: [_ w435] -> w430
                          frame "氨氮、总磷总氮", Default {
                          }
                          frame "氨氮总磷" {
                            n203 = call "取水点无水样数据存储.vi"("error in (no error)"=w438, "数据标识"=w436, "数据类型"=w437, "table"="总磷") -> ("error out"=w435:errorcluster)  [unwired: 7 in]
                          }
                        }
                      }
                    }
                    n204 = case shown="真" w359 {
                      tunnel: w358 -> [_ w368]
                      tunnel: w357 -> [_ w369]
                      tunnel: [_ w367] -> _
                      frame False {
                      }
                      frame True {
                        n205 = global read "系统设置全局变量.vi" "营养盐类型"() -> (w366:enum16{"氨氮、总磷总氮", "氨氮总磷", "氨氮、总磷、总氮"})
                        n206 = case shown="\"氨氮、总磷、总氮\"" w366 {
                          tunnel: w369 -> [_ w372]
                          tunnel: w368 -> [_ w371]
                          tunnel: [_ w370] -> w367
                          frame "氨氮、总磷总氮", Default {
                          }
                          frame "氨氮、总磷、总氮" {
                            n207 = call "取水点无水样数据存储.vi"("数据标识"=w372, "数据类型"=w371, "table"="总氮") -> ("error out"=w370:errorcluster)  [unwired: 8 in]
                          }
                        }
                      }
                    }
                    n208 = case shown="真" w363 {
                      tunnel: w358 -> [_ w427]
                      tunnel: [_ w426] -> _
                      tunnel: w357 -> [_ w425]
                      frame False {
                      }
                      frame True {
                        n209 = call "取水点无水样数据存储.vi"("数据标识"=w425, "数据类型"=w427, "table"="CODMn") -> ("error out"=w426:errorcluster)  [unwired: 8 in]
                      }
                    }
                    n210 = case shown="真" w362 {
                      tunnel: w358 -> [_ w423]
                      tunnel: [_ w422] -> _
                      tunnel: w357 -> [_ w421]
                      frame False {
                      }
                      frame True {
                        n211 = call "取水点无水样数据存储.vi"("数据标识"=w421, "数据类型"=w423, "table"="CODCr") -> ("error out"=w422:errorcluster)  [unwired: 8 in]
                      }
                    }
                    n212 = case shown="真" w360 {
                      tunnel: w358 -> [_ w376]
                      tunnel: [_ w377] -> _
                      tunnel: w357 -> [_ w375]
                      frame False {
                      }
                      frame True {
                        n213 = global read "系统设置全局变量.vi" "营养盐类型"() -> (w374:enum16{"氨氮、总磷总氮", "氨氮总磷", "氨氮、总磷、总氮"})
                        n214 = case shown="\"氨氮总磷\", 默认" w374 {
                          tunnel: [w382 _] -> w378
                          tunnel: w375 -> [w381 _]
                          tunnel: w376 -> [w380 _]
                          frame "氨氮、总磷总氮" {
                            n215 = call "取水点无水样数据存储.vi"("数据标识"=w381, "数据类型"=w380, "table"="总氮") -> ("error out"=w382:errorcluster)  [unwired: 8 in]
                          }
                          frame "氨氮总磷", Default {
                          }
                        }
                        n216 = call "取水点无水样数据存储.vi"("error in (no error)"=w378, "数据标识"=w375, "数据类型"=w376, "table"="总磷") -> ("error out"=w377:errorcluster)  [unwired: 7 in]
                      }
                    }
                    n217 = case shown="真" w356 {
                      tunnel: w358 -> [_ w392]
                      tunnel: w357 -> [_ w384]
                      frame False {
                      }
                      frame True {
                        n218 = global read "断电保存变量.vi" "pH"() -> (w390:bool)
                        n219 = global read "断电保存变量.vi" "DO"() -> (w389:bool)
                        n220 = global read "断电保存变量.vi" "Turb"() -> (w388:bool)
                        n221 = global read "断电保存变量.vi" "Temp"() -> (w391:bool)
                        n222 = global read "断电保存变量.vi" "Cond"() -> (w387:bool)
                        n223 = global read "断电保存变量.vi" "藻密度"() -> (w385:bool)
                        n224 = global read "断电保存变量.vi" "叶绿素a启用"() -> (w386:bool)
                        n225 = case shown="真" w390 {
                          tunnel: w392 -> [_ w415]
                          tunnel: [_ w414] -> _
                          tunnel: w384 -> [_ w413]
                          frame False {
                          }
                          frame True {
                            n226 = call "取水点无水样数据存储.vi"("数据标识"=w413, "数据类型"=w415, "table"="pH") -> ("error out"=w414:errorcluster)  [unwired: 8 in]
                          }
                        }
                        n227 = case shown="真" w389 {
                          tunnel: w392 -> [_ w411]
                          tunnel: [_ w410] -> _
                          tunnel: w384 -> [_ w409]
                          frame False {
                          }
                          frame True {
                            n228 = call "取水点无水样数据存储.vi"("数据标识"=w409, "数据类型"=w411, "table"="DO") -> ("error out"=w410:errorcluster)  [unwired: 8 in]
                          }
                        }
                        n229 = case shown="真" w388 {
                          tunnel: w392 -> [_ w403]
                          tunnel: [_ w402] -> _
                          tunnel: w384 -> [_ w401]
                          frame False {
                          }
                          frame True {
                            n230 = call "取水点无水样数据存储.vi"("数据标识"=w401, "数据类型"=w403, "table"="浊度") -> ("error out"=w402:errorcluster)  [unwired: 8 in]
                          }
                        }
                        n231 = case shown="真" w391 {
                          tunnel: w392 -> [_ w419]
                          tunnel: [_ w418] -> _
                          tunnel: w384 -> [_ w417]
                          frame False {
                          }
                          frame True {
                            n232 = call "取水点无水样数据存储.vi"("数据标识"=w417, "数据类型"=w419, "table"="水温") -> ("error out"=w418:errorcluster)  [unwired: 8 in]
                          }
                        }
                        n233 = case shown="真" w387 {
                          tunnel: w392 -> [_ w407]
                          tunnel: [_ w406] -> _
                          tunnel: w384 -> [_ w405]
                          frame False {
                          }
                          frame True {
                            n234 = call "取水点无水样数据存储.vi"("数据标识"=w405, "数据类型"=w407, "table"="电导率") -> ("error out"=w406:errorcluster)  [unwired: 8 in]
                          }
                        }
                        n235 = case shown="真" w385 {
                          tunnel: w392 -> [_ w395]
                          tunnel: [_ w394] -> _
                          tunnel: w384 -> [_ w393]
                          frame False {
                          }
                          frame True {
                            n236 = call "取水点无水样数据存储.vi"("数据标识"=w393, "数据类型"=w395, "table"="藻密度") -> ("error out"=w394:errorcluster)  [unwired: 8 in]
                          }
                        }
                        n237 = case shown="真" w386 {
                          tunnel: w392 -> [_ w399]
                          tunnel: [_ w398] -> _
                          tunnel: w384 -> [_ w397]
                          frame False {
                          }
                          frame True {
                            n238 = call "取水点无水样数据存储.vi"("数据标识"=w397, "数据类型"=w399, "table"="叶绿素a") -> ("error out"=w398:errorcluster)  [unwired: 8 in]
                          }
                        }
                      }
                    }
                  }
                }
              }
              frame "集成干预" {
                n239 = Unbundle By Name(w447) -> ("氨氮"=w446:bool, "CODMn"=w445:bool, "CODcr"=w444:bool, "多参数"=w443:bool, "总磷总氮"=w442:bool, "总氮"=w440:bool)
                n240 = case shown="真" w446 {
                  tunnel: w441 -> [_ w526]
                  frame False {
                  }
                  frame True {
                    n241 = call "获取最近两组水样测试数据.vi"("运行模式"=w526, "table"="氨氮") -> ("error out"=w527:errorcluster, "存储变量"=w528:T16)  [unwired: 8 in]
                    n242 = call "集成干预测试数据存储.vi"("error in (no error)"=w527, "存储变量"=w528) -> ()  [unwired: 9 in, 1 out]
                  }
                }
                n243 = case shown="真" w440 {
                  tunnel: w441 -> [_ w448]
                  frame False {
                  }
                  frame True {
                    n244 = call "获取最近两组水样测试数据.vi"("运行模式"=w448, "table"="总氮") -> ("error out"=w451:errorcluster, "存储变量"=w450:T16)  [unwired: 8 in]
                    n245 = call "集成干预测试数据存储.vi"("error in (no error)"=w451, "存储变量"=w450) -> ()  [unwired: 9 in, 1 out]
                  }
                }
                n246 = case shown="真" w445 {
                  tunnel: w441 -> [_ w522]
                  frame False {
                  }
                  frame True {
                    n247 = call "获取最近两组水样测试数据.vi"("运行模式"=w522, "table"="CODMn") -> ("error out"=w523:errorcluster, "存储变量"=w524:T16)  [unwired: 8 in]
                    n248 = call "集成干预测试数据存储.vi"("error in (no error)"=w523, "存储变量"=w524) -> ()  [unwired: 9 in, 1 out]
                  }
                }
                n249 = case shown="真" w444 {
                  tunnel: w441 -> [_ w518]
                  frame False {
                  }
                  frame True {
                    n250 = call "获取最近两组水样测试数据.vi"("运行模式"=w518, "table"="CODCr") -> ("error out"=w519:errorcluster, "存储变量"=w520:T16)  [unwired: 8 in]
                    n251 = call "集成干预测试数据存储.vi"("error in (no error)"=w519, "存储变量"=w520) -> ()  [unwired: 9 in, 1 out]
                  }
                }
                n252 = case shown="真" w442 {
                  tunnel: w441 -> [_ w453]
                  frame False {
                  }
                  frame True {
                    n253 = call "获取最近两组水样测试数据.vi"("运行模式"=w453, "table"="总磷") -> ("error out"=w455:errorcluster, "存储变量"=w456:T16)  [unwired: 8 in]
                    n254 = call "集成干预测试数据存储.vi"("error in (no error)"=w455, "存储变量"=w456) -> ("error out"=w454:errorcluster)  [unwired: 9 in]
                    n255 = global read "系统设置全局变量.vi" "总氮启用"() -> (w452:bool)
                    n256 = case shown="真" w452 {
                      tunnel: w454 -> [_ w459]
                      tunnel: w453 -> [_ w458]
                      frame False {
                      }
                      frame True {
                        n257 = call "获取最近两组水样测试数据.vi"("error in (no error)"=w459, "运行模式"=w458, "table"="总氮") -> ("error out"=w462:errorcluster, "存储变量"=w461:T16)  [unwired: 7 in]
                        n258 = call "集成干预测试数据存储.vi"("error in (no error)"=w462, "存储变量"=w461) -> ()  [unwired: 9 in, 1 out]
                      }
                    }
                  }
                }
                n259 = case shown="真" w443 {
                  tunnel: w441 -> [_ w463]
                  frame False {
                  }
                  frame True {
                    n260 = global read "断电保存变量.vi" "Temp"() -> (w470:bool)
                    n261 = case shown="真" w470 {
                      tunnel: [_ w514] -> w476
                      tunnel: w463 -> [_ w513]
                      frame False {
                      }
                      frame True {
                        n262 = call "获取最近两组水样测试数据.vi"("运行模式"=w513, "table"="水温") -> ("error out"=w517:errorcluster, "存储变量"=w516:T16)  [unwired: 8 in]
                        n263 = call "集成干预测试数据存储.vi"("error in (no error)"=w517, "存储变量"=w516) -> ("error out"=w514:errorcluster)  [unwired: 9 in]
                      }
                    }
                    n264 = global read "断电保存变量.vi" "pH"() -> (w469:bool)
                    n265 = case shown="真" w469 {
                      tunnel: [_ w509] -> w475
                      tunnel: w476 -> [_ w508]
                      tunnel: w463 -> [_ w507]
                      frame False {
                      }
                      frame True {
                        n266 = call "获取最近两组水样测试数据.vi"("error in (no error)"=w508, "运行模式"=w507, "table"="pH") -> ("error out"=w512:errorcluster, "存储变量"=w511:T16)  [unwired: 7 in]
                        n267 = call "集成干预测试数据存储.vi"("error in (no error)"=w512, "存储变量"=w511) -> ("error out"=w509:errorcluster)  [unwired: 9 in]
                      }
                    }
                    n268 = global read "断电保存变量.vi" "DO"() -> (w468:bool)
                    n269 = case shown="真" w468 {
                      tunnel: [_ w503] -> w474
                      tunnel: w475 -> [_ w502]
                      tunnel: w463 -> [_ w501]
                      frame False {
                      }
                      frame True {
                        n270 = call "获取最近两组水样测试数据.vi"("error in (no error)"=w502, "运行模式"=w501, "table"="DO") -> ("error out"=w506:errorcluster, "存储变量"=w505:T16)  [unwired: 7 in]
                        n271 = call "集成干预测试数据存储.vi"("error in (no error)"=w506, "存储变量"=w505) -> ("error out"=w503:errorcluster)  [unwired: 9 in]
                      }
                    }
                    n272 = global read "断电保存变量.vi" "Cond"() -> (w467:bool)
                    n273 = case shown="真" w467 {
                      tunnel: [_ w497] -> w473
                      tunnel: w474 -> [_ w496]
                      tunnel: w463 -> [_ w495]
                      frame False {
                      }
                      frame True {
                        n274 = call "获取最近两组水样测试数据.vi"("error in (no error)"=w496, "运行模式"=w495, "table"="电导率") -> ("error out"=w500:errorcluster, "存储变量"=w499:T16)  [unwired: 7 in]
                        n275 = call "集成干预测试数据存储.vi"("error in (no error)"=w500, "存储变量"=w499) -> ("error out"=w497:errorcluster)  [unwired: 9 in]
                      }
                    }
                    n276 = global read "断电保存变量.vi" "Turb"() -> (w466:bool)
                    n277 = case shown="真" w466 {
                      tunnel: [_ w491] -> w472
                      tunnel: w473 -> [_ w490]
                      tunnel: w463 -> [_ w489]
                      frame False {
                      }
                      frame True {
                        n278 = call "获取最近两组水样测试数据.vi"("error in (no error)"=w490, "运行模式"=w489, "table"="浊度") -> ("error out"=w494:errorcluster, "存储变量"=w493:T16)  [unwired: 7 in]
                        n279 = call "集成干预测试数据存储.vi"("error in (no error)"=w494, "存储变量"=w493) -> ("error out"=w491:errorcluster)  [unwired: 9 in]
                      }
                    }
                    n280 = global read "断电保存变量.vi" "叶绿素a启用"() -> (w465:bool)
                    n281 = case shown="真" w465 {
                      tunnel: [_ w485] -> w471
                      tunnel: w472 -> [_ w484]
                      tunnel: w463 -> [_ w483]
                      frame False {
                      }
                      frame True {
                        n282 = call "获取最近两组水样测试数据.vi"("error in (no error)"=w484, "运行模式"=w483, "table"="叶绿素a") -> ("error out"=w488:errorcluster, "存储变量"=w487:T16)  [unwired: 7 in]
                        n283 = call "集成干预测试数据存储.vi"("error in (no error)"=w488, "存储变量"=w487) -> ("error out"=w485:errorcluster)  [unwired: 9 in]
                      }
                    }
                    n284 = global read "断电保存变量.vi" "藻密度"() -> (w464:bool)
                    n285 = case shown="真" w464 {
                      tunnel: [_ w479] -> _
                      tunnel: w471 -> [_ w478]
                      tunnel: w463 -> [_ w477]
                      frame False {
                      }
                      frame True {
                        n286 = call "获取最近两组水样测试数据.vi"("error in (no error)"=w478, "运行模式"=w477, "table"="藻密度") -> ("error out"=w482:errorcluster, "存储变量"=w481:T16)  [unwired: 7 in]
                        n287 = call "集成干预测试数据存储.vi"("error in (no error)"=w482, "存储变量"=w481) -> ("error out"=w479:errorcluster)  [unwired: 9 in]
                      }
                    }
                  }
                }
              }
            }
          }
        }
        n288 = Unbundle By Name(w323) -> ("R0"=w322:i16)
        n289 = Equal To 0?(x=w322) -> (x = 0?=w321:bool)
        n290 = Select(t=enum16{"初始化", "采配水启动", "仪器操作", "反冲洗", "结束"}."结束" ("枚举"), s=w321, f=enum16{"初始化", "采配水启动", "仪器操作", "反冲洗", "结束"}."反冲洗" ("枚举")) -> (s? t:f=w318:enum16{"初始化", "采配水启动", "仪器操作", "反冲洗", "结束"})
      }
      frame "结束" {
        n291 = Release Queue(queue=w534) -> ()  [unwired: 2 in, 3 out]
        n292 = Unbundle By Name(w531) -> ("测试模式"=w532:enum16{"正常测试", "集成干预"})
        n293 = Cancel Notification(0:w535) -> (8:w536:refnum<notifier>)  [unwired: 1 in, 2 out]
        n294 = case shown="\"集成干预\"" w532 {
          tunnel: w530 -> [_ w539]
          frame "正常测试", Default {
          }
          frame "集成干预" {
            n295 = global write "系统设置全局变量.vi" "运行模式"(w539) -> ()
          }
        }
        n296 = Release Notifier(notifier=w536) -> ()  [unwired: 2 in, 3 out]
      }
    }
    n297 = Wait (ms)(milliseconds to wait=u32 1000 ("等待时间（毫秒）")) -> ()  [unwired: 1 out]
    n298 = Format Into String(format string="%s,当前运行时间%d秒" ("格式字符串"), w15, w11) -> (resulting string=w16:string)  [unwired: 2 in, 1 out]
    n299 = global write "采配水全局变量.vi" "运行状态显示"(w16) -> ()
  }
